vi "Write Device Icon Name.vi"(8 "error in (no error)":errorcluster, 10 "Device Icon Name":string[](array[string]), 11 "Device Configuration in":refnum<class "Device Configuration.lvclass">) -> (0 "error out":errorcluster, 3 "Device Configuration out":refnum<class "Device Configuration.lvclass">)   [LabVIEW 2014, in "Device Configuration.lvclass"]
uses:
  Device Configuration.lvclass
  Device Configuration.lvclass/Device Configuration.ctl
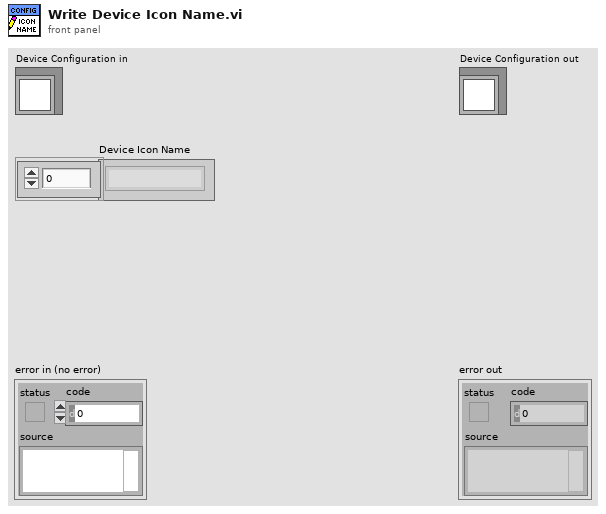
[diagram p1: front panel]
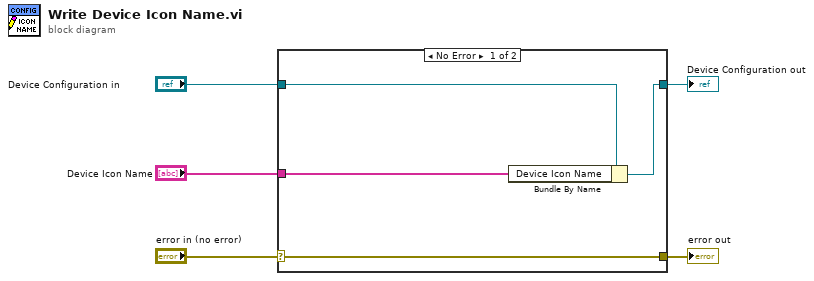
[diagram p0: block diagram]
diagram:
  n1 = case shown="No Error" "error in (no error)" {
    selector: "error in (no error)" -> [w9 w10]
    tunnel: [w9 w10] -> w4
    tunnel: [w7 w11] -> w2
    tunnel: "Device Configuration in" -> [w8 w11]
    tunnel: "Device Icon Name" -> [w6 _]
    frame No Error {
      n2 = Bundle By Name(cluster=w8, "Device Icon Name"=w6) -> (w7:refnum<class "Device Configuration.lvclass">)
    }
    frame Error {
    }
  }
  "error out" <- w4
  "Device Configuration out" <- w2
